vi "Integral x(t).vi"(6 "integration method":T1=1 items=["Trapezoidal Rule", "Simpson's Rule", "Simpson's 3/8 Rule", "Bode Rule"], 8 "dt":dbl=1.0, 9 "Final Condition":dbl[](array[numeric])=[0.0], 10 "Initial Condition":dbl[](array[numeric])=[0.0], 11 "X":dbl[](array[numeric])) -> (0 "error":i32, 3 "Integral X":dbl[](array[numeric]))   [LabVIEW 2018, in "NI_AALPro.lvlib"]
doc: "Performs the discrete integration of the sampled signal <B>X</B>."
uses:
  NI_AALPro.lvlib
  Integral Method.ctl
  <resource>/lvanlys.dll
panel:
  # "Integral x(t)"
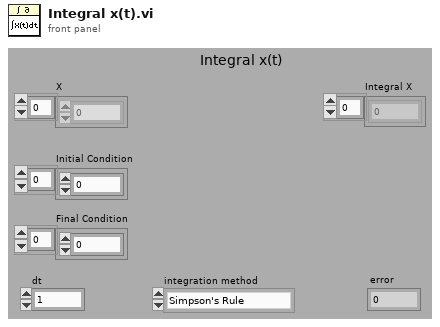
[diagram p1: front panel]
types:
  T1 = typedef "NI_AALPro.lvlib/Integral Method.ctl" = i32
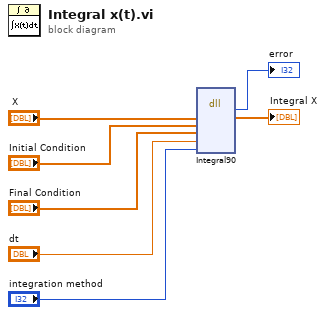
[diagram p0: block diagram]
diagram:
  n1 = dll-call lib="C:/Program Files (x86)/National Instruments/LabVIEW 2018/resource/lvanlys.*" fn="Integral90"("X"="X", "initial condition"="Initial Condition", "final condition"="Final Condition", "dt"="dt", "method"="integration method") -> ("error"=→"error":i32, "X"=→"Integral X":dbl[])  [unwired: 7 in, 2 out]
